vi "Add Version Element to Map.vi"(9 "Version":i32[](array[numeric]), 10 "Package Name":string, 11 "Version map in":map{string, i32[]}(c390)) -> (3 "Version map out":map{string, i32[]}(c390))   [LabVIEW 2019, in "Project.Dependencies Finder.lvlib" / "Dependency Source_VIPM.lvclass"]
doc: "Add a version element to the version map if the version is new or higher than the previous stored version."
uses:
  Dependency Source_VIPM.lvclass
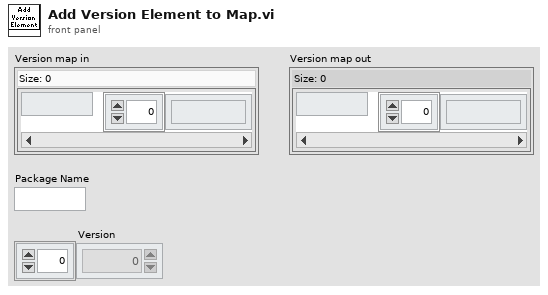
[diagram p1: front panel]
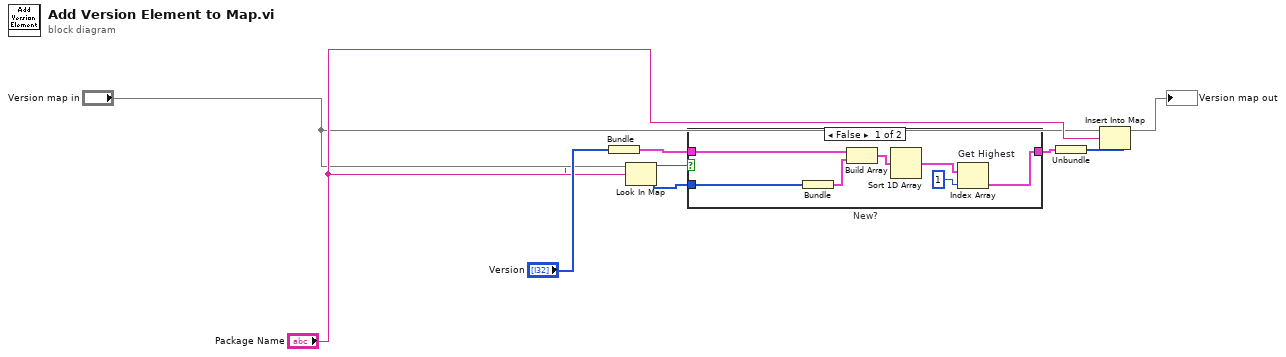
[diagram p0: block diagram]
diagram:
  n1 = Bundle("Version"="Version") -> (w8:cluster{"Version":i32[]})  [unwired: 1 in]
  n2 = Look In Map(map="Version map in", key="Package Name") -> (key not found?=w1:bool, value=w4:i32[])  [unwired: 1 in]
  n3 = case "New?" shown="False" w1 {
    tunnel: w4 -> [w16 _]
    tunnel: [w11 w17] -> w6
    tunnel: w8 -> [w10 w17]
    frame False {
      n4 = Bundle("value"=w16) -> (w15:cluster{"value":i32[]})  [unwired: 1 in]
      n5 = Build Array(w10, w15) -> (w14:cluster{"value":i32[]}[])
      n6 = Sort 1D Array(array=w14) -> (sorted array=w13:cluster{"value":i32[]}[])
      n7 = Index Array "Get Highest"(array=w13, index=1) -> (element=w11:cluster{"value":i32[]})
    }
    frame True {
    }
  }
  n8 = Unbundle(w6) -> ("Version"=w7:i32[])
  n9 = Insert Into Map(map in="Version map in", key="Package Name", value=w7) -> (map out=→"Version map out":map{string, i32[]})  [unwired: 2 out]
